vi "AdquisicioDadesYoctopuce.vi"(1 "HardName":refnum<vi>, 5 "online?":refnum<vi>, 7 "AssaigActiu":refnum<vi>, 8 "Stop":refnum<vi>, 10 "Temperature name":string="THRMCPL1-204875.temperature1", 11 "user event in":refnum<user-event>) -> (0 "error out":errorcluster, 3 "isOnline 2":bool)   [LabVIEW 2017]
panel:
  out "error msg":string
  out "Temp":dbl
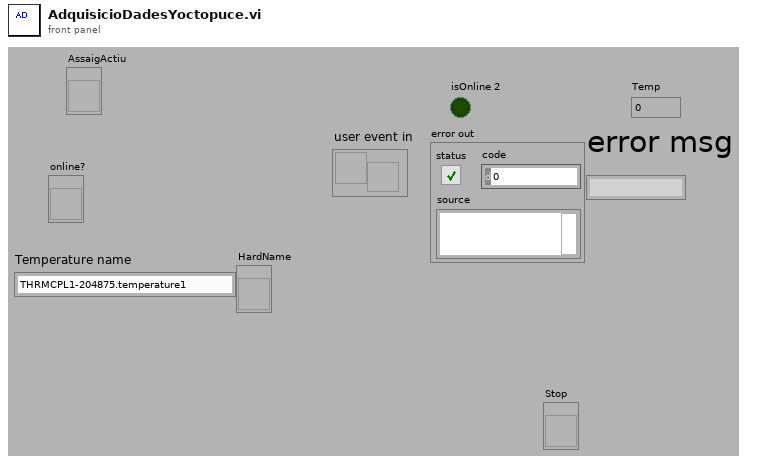
[diagram p1: front panel]
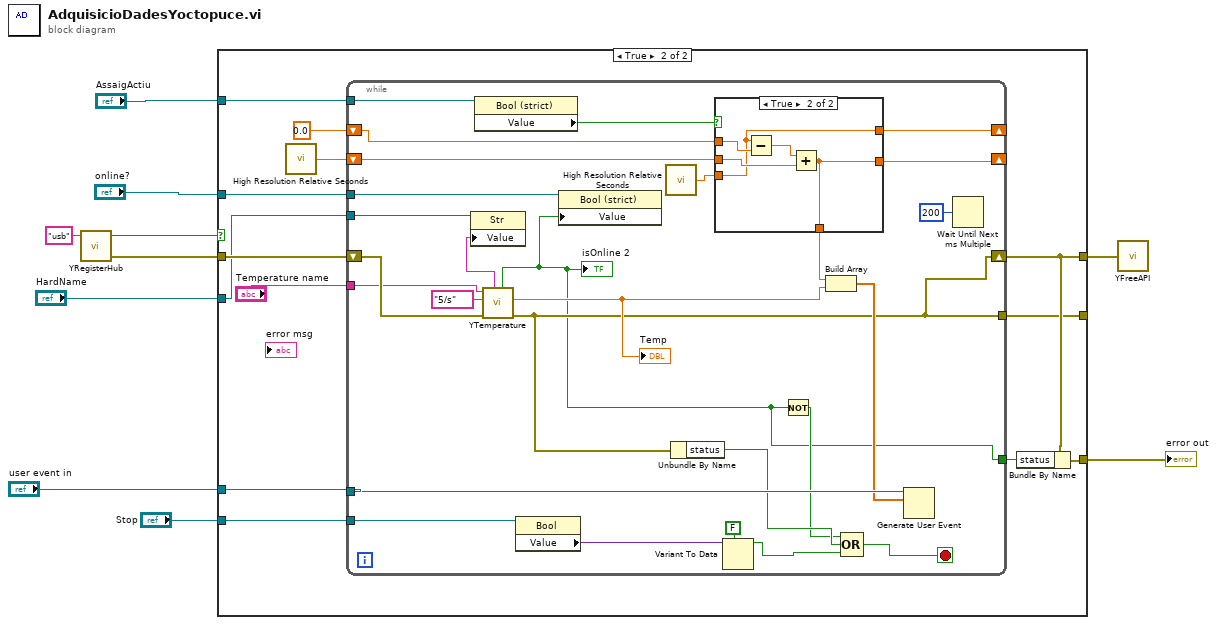
[diagram p0: block diagram]
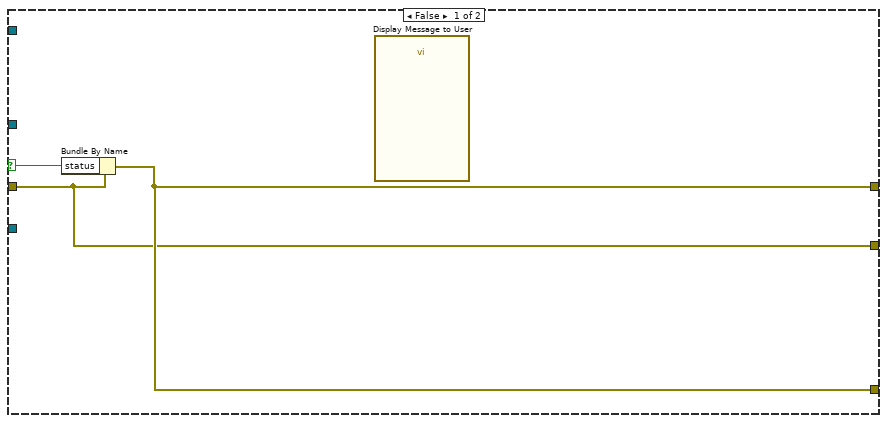
[diagram p2: hidden frame]
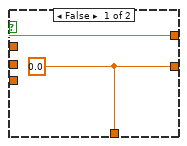
[diagram p3: hidden frame]
diagram:
  n1 = call "YRegisterHub.vi"("url"="usb") -> ("error out"=w9:errorcluster, "success"=w6:bool)  [unwired: 2 in, 1 out]
  n2 = case shown="True" w6 {
    selector: w6 -> [w12 _]
    tunnel: "Stop" -> [_ w26]
    tunnel: w9 -> [w11 w24]
    tunnel: [w13 w17] -> w5
    tunnel: "user event in" -> [_ w25]
    tunnel: [w13 w19] -> w4
    tunnel: "AssaigActiu" -> [_ w23]
    tunnel: [w11 w16] -> _
    tunnel: "online?" -> [_ w15]
    tunnel: "HardName" -> [_ w14]
    frame False {
      n3 = Bundle By Name(cluster=w11, "status"=w12) -> (w13:errorcluster)
      n4 = call "Display Message to User"() -> ()  [unwired: 10 in, 2 out]
    }
    frame True {
      n5 = call <vilib>:"High Resolution Relative Seconds.vi"() -> ("relative seconds"=w21:dbl)
      n6 = while {
        tunnel: w26 -> [w53]
        tunnel: w25 -> [w50]
        shift-right: [w31] -> w17
        shift-left: w24 -> [w40]
        tunnel: w23 -> [w46]
        shift-right: [w41] -> _
        shift-left: 0.0 ("relative seconds") -> [w43]
        shift-right: [w42] -> _
        shift-left: w21 -> [w45]
        tunnel: "Temperature name" -> [w38]
        tunnel: [w29] -> w18
        tunnel: [w31] -> w16
        tunnel: w15 -> [w30]
        tunnel: w14 -> [w28]
        stop <- w33 stop-if-true
        n7 = property class="Bool (strict)"(reference=w46) -> ("Value"=w47:bool)  [unwired: 1 in, 2 out]
        n8 = call "YTemperature.vi"("error in (no error)"=w40, "reportFrequency in"="5/s", "Temperature name"=w38) -> ("error out"=w31:errorcluster, "currentValue out"=w36:dbl, "isOnline"=w29:bool, "hardware name"=w27:string)  [unwired: 3 in, 2 out]
        "Temp" <- w36
        "isOnline 2" <- w29
        n9 = property class="Str"(reference=w28, "Value"=w27) -> ()  [unwired: 1 in, 2 out]
        n10 = property class="Bool"(reference=w53) -> ("Value"=w52:variant)  [unwired: 1 in, 2 out]
        n11 = property class="Bool (strict)"(reference=w30, "Value"=w29) -> ()  [unwired: 1 in, 2 out]
        n12 = call <vilib>:"High Resolution Relative Seconds.vi"() -> ("relative seconds"=w44:dbl)
        n13 = Unbundle By Name(w31) -> ("status"=w35:bool)
        n14 = case shown="True" w47 {
          tunnel: w45 -> [_ w59]
          tunnel: w44 -> [w55 w56]
          tunnel: w43 -> [_ w58]
          tunnel: [w54 w57] -> w37
          tunnel: [w54 w57] -> w42
          tunnel: [w55 w56] -> w41
          frame False {
            w54 = 0.0
          }
          frame True {
            n15 = Subtract(x=w56, y=w58) -> (x-y=w60:dbl)
            n16 = Add(x=w60, y=w59) -> (x+y=w57:dbl)
          }
        }
        n17 = Variant To Data(type=FALSE, Variant=w52) -> (data=w34:bool)  [unwired: 1 in, 1 out]
        n18 = Not(x=w29) -> (.not. x?=w32:bool)
        n19 = Build Array(w37, w36) -> (w49:dbl[])
        n20 = Compound Arithmetic op=OR(w32, w35, w34) -> (w33:bool)
        n21 = Generate User Event(user event=w50, event data cluster=w49) -> ()  [unwired: 2 in, 2 out]
        n22 = Wait Until Next ms Multiple(millisecond multiple=u32 200) -> ()  [unwired: 1 out]
      }
      n23 = Bundle By Name(cluster=w17, "status"=w18) -> (w19:errorcluster)
    }
  }
  "error out" <- w4
  n24 = call "YFreeAPI.vi"("error in (no error)"=w5) -> ()  [unwired: 1 out]
